vi "Calculadora.vi"() -> ()   [LabVIEW 2020]
panel:
  out "Valor 2\nNegativo":bool
  out "Valor 1 \nNegativo":bool
  in  "Finalizar":bool
  in  "Un solo valor":T1(ring)
  in  "Dos valores":T2(ring)
  in  "¿Con que se \ndesea trabajar?":u16(ring) items=["Dos valores", "Valor 1", "Valor 2"]
  out "Resultado":dbl
  in  "Valor 2":dbl
  in  "Valor 1":dbl
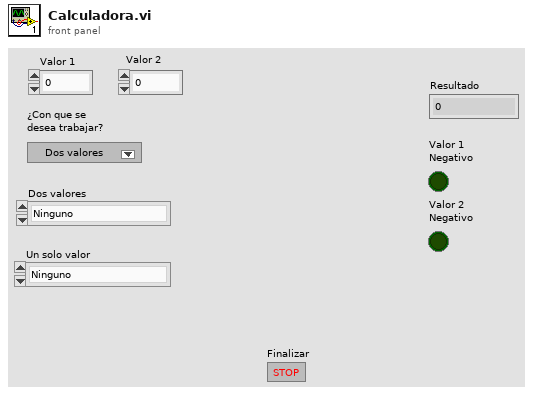
[diagram p1: front panel]
types:
  T1 = enum16{"Ninguno", "Potencia Cuadrada", "Raiz Cuadrada", "Seno", "Coseno", "Tangente", "Grados --> Radianes"}
  T2 = enum16{"Ninguno", "Suma", "Resta", "Multiplicación", "División", "Valor 1 elevado a Valor 2", "Valor 2 elevado a Valor 1"}
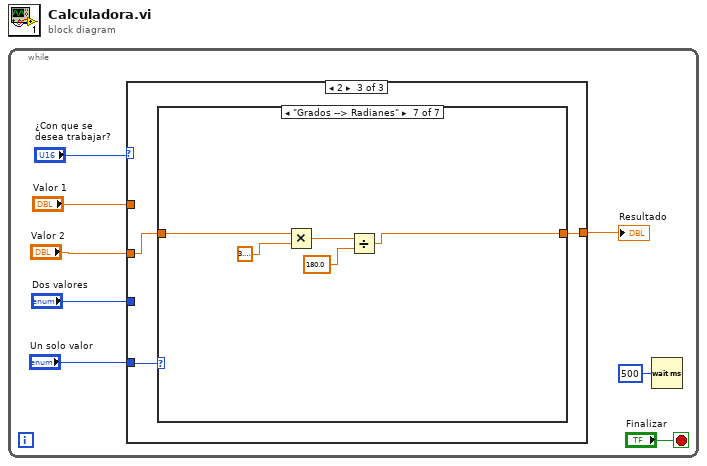
[diagram p0: block diagram]
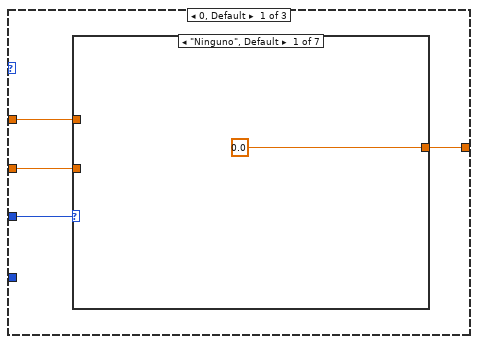
[diagram p2: hidden frame]
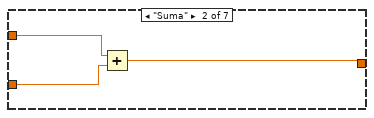
[diagram p3: hidden frame]
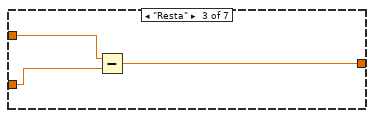
[diagram p4: hidden frame]
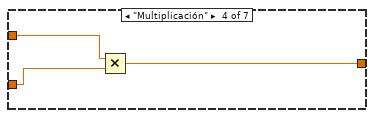
[diagram p5: hidden frame]
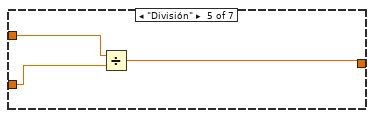
[diagram p6: hidden frame]
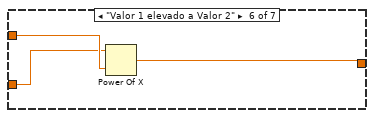
[diagram p7: hidden frame]
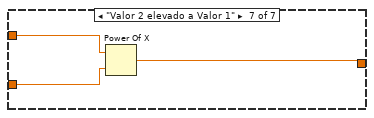
[diagram p8: hidden frame]
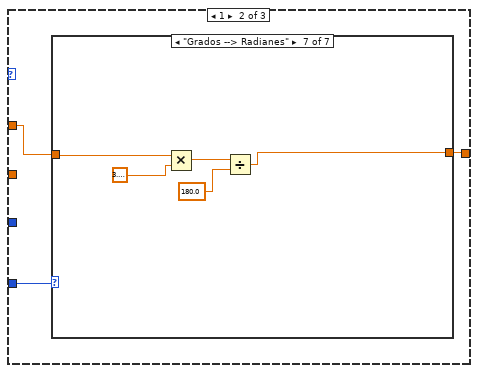
[diagram p9: hidden frame]
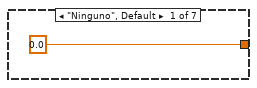
[diagram p10: hidden frame]
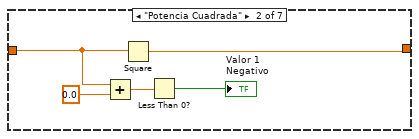
[diagram p11: hidden frame]
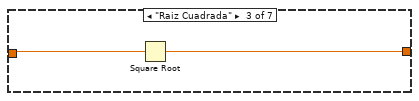
[diagram p12: hidden frame]
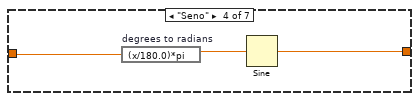
[diagram p13: hidden frame]
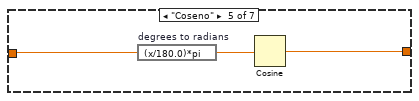
[diagram p14: hidden frame]
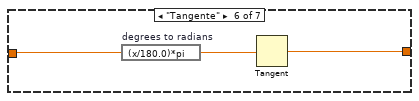
[diagram p15: hidden frame]
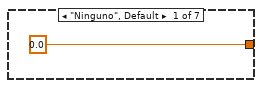
[diagram p16: hidden frame]
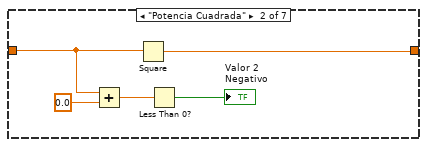
[diagram p17: hidden frame]
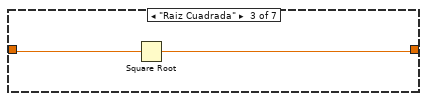
[diagram p18: hidden frame]
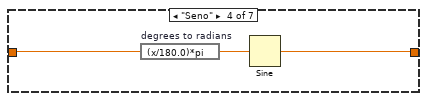
[diagram p19: hidden frame]
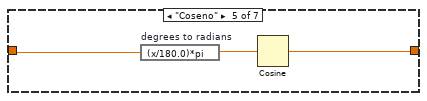
[diagram p20: hidden frame]
diagram:
  n1 = while {
    stop <- "Finalizar" stop-if-true
    n2 = case shown="2" "¿Con que se \ndesea trabajar?" {
      tunnel: "Dos valores" -> [w12 _ _]
      tunnel: [w11 w33 w58] -> w4
      tunnel: "Valor 1" -> [w10 w32 _]
      tunnel: "Valor 2" -> [w9 _ w57]
      tunnel: "Un solo valor" -> [_ w34 w59]
      frame 0, Default {
        n3 = case shown="\"Ninguno\", Default" w12 {
          tunnel: [0.0 w16 w19 w22 w25 w28 w31] -> w11
          tunnel: w10 -> [_ w15 w18 w21 w24 w27 w30]
          tunnel: w9 -> [_ w14 w17 w20 w23 w26 w29]
          frame "Ninguno", Default {
          }
          frame "Suma" {
            n4 = Add(x=w15, y=w14) -> (x+y=w16:dbl)
          }
          frame "Resta" {
            n5 = Subtract(x=w18, y=w17) -> (x-y=w19:dbl)
          }
          frame "Multiplicación" {
            n6 = Multiply(x=w21, y=w20) -> (x*y=w22:dbl)
          }
          frame "División" {
            n7 = Divide(x=w24, y=w23) -> (x/y=w25:dbl)
          }
          frame "Valor 1 elevado a Valor 2" {
            n8 = Power Of X(1:w27, 2:w26) -> (0:w28:dbl)
          }
          frame "Valor 2 elevado a Valor 1" {
            n9 = Power Of X(1:w29, 2:w30) -> (0:w31:dbl)
          }
        }
      }
      frame 1 {
        n10 = case shown="\"Grados --> Radianes\"" w34 {
          tunnel: [0.0 w40 w42 w45 w48 w51 w52] -> w33
          tunnel: w32 -> [_ w39 w41 w43 w46 w49 w56]
          frame "Ninguno", Default {
          }
          frame "Potencia Cuadrada" {
            n11 = Add(x=w39, y=0.0) -> (x+y=w37:dbl)
            n12 = Square(x=w39) -> (x^2=w40:dbl)
            n13 = Less Than 0?(x=w37) -> (x < 0?=→"Valor 1 \nNegativo":bool)
          }
          frame "Raiz Cuadrada" {
            n14 = Square Root(x=w41) -> (sqrt(x)=w42:dbl)
          }
          frame "Seno" {
            n15 = expression code="(x/180.0)*pi" "degrees to radians"(w43) -> (w44:dbl)
            n16 = Sine(x=w44) -> (sin(x)=w45:dbl)
          }
          frame "Coseno" {
            n17 = expression code="(x/180.0)*pi" "degrees to radians"(w46) -> (w47:dbl)
            n18 = Cosine(x=w47) -> (cos(x)=w48:dbl)
          }
          frame "Tangente" {
            n19 = expression code="(x/180.0)*pi" "degrees to radians"(w49) -> (w50:dbl)
            n20 = Tangent(1:w50) -> (0:w51:dbl)
          }
          frame "Grados --> Radianes" {
            n21 = Multiply(x=w56, y=3.141592653589793) -> (x*y=w54:dbl)
            n22 = Divide(x=w54, y=180.0) -> (x/y=w52:dbl)
          }
        }
      }
      frame 2 {
        n23 = case shown="\"Grados --> Radianes\"" w59 {
          tunnel: [0.0 w65 w67 w70 w73 w76 w77] -> w58
          tunnel: w57 -> [_ w64 w66 w68 w71 w74 w81]
          frame "Ninguno", Default {
          }
          frame "Potencia Cuadrada" {
            n24 = Add(x=w64, y=0.0) -> (x+y=w62:dbl)
            n25 = Square(x=w64) -> (x^2=w65:dbl)
            n26 = Less Than 0?(x=w62) -> (x < 0?=→"Valor 2\nNegativo":bool)
          }
          frame "Raiz Cuadrada" {
            n27 = Square Root(x=w66) -> (sqrt(x)=w67:dbl)
          }
          frame "Seno" {
            n28 = expression code="(x/180.0)*pi" "degrees to radians"(w68) -> (w69:dbl)
            n29 = Sine(x=w69) -> (sin(x)=w70:dbl)
          }
          frame "Coseno" {
            n30 = expression code="(x/180.0)*pi" "degrees to radians"(w71) -> (w72:dbl)
            n31 = Cosine(x=w72) -> (cos(x)=w73:dbl)
          }
          frame "Tangente" {
            n32 = expression code="(x/180.0)*pi" "degrees to radians"(w74) -> (w75:dbl)
            n33 = Tangent(1:w75) -> (0:w76:dbl)
          }
          frame "Grados --> Radianes" {
            n34 = Multiply(x=w81, y=3.141592653589793) -> (x*y=w79:dbl)
            n35 = Divide(x=w79, y=180.0) -> (x/y=w77:dbl)
          }
        }
      }
    }
    "Resultado" <- w4
    n36 = Wait (ms)(milliseconds to wait=u32 500) -> ()  [unwired: 1 out]
  }
